vi "nodeInfo.get_OS.vi"(5 "error in (no error)":errorcluster) -> (16 "OS":string, 19 "error out":errorcluster)   [LabVIEW 2014, in "LVNodeInfo.lvlib"]
doc: "Gets the name of the operating system."
uses:
  LVNodeInfo.lvlib
  NodeMon/bin/libNodeInfo.dll
  NodeMon/bin/libNodeInfo.so
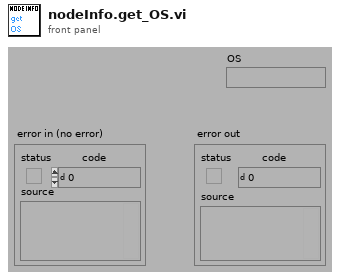
[diagram p1: front panel]
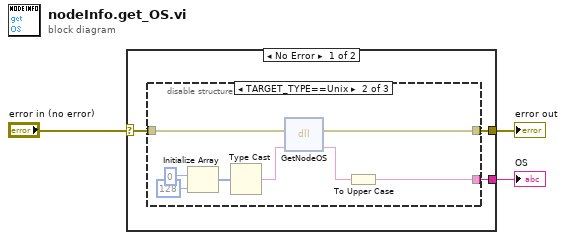
[diagram p0: block diagram]
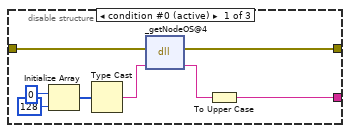
[diagram p2: hidden frame]
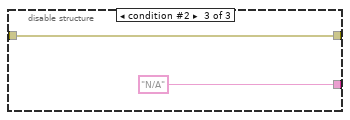
[diagram p3: hidden frame]
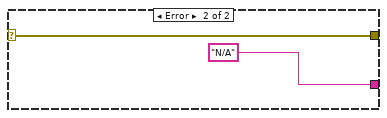
[diagram p4: hidden frame]
diagram:
  n1 = case shown="No Error" "error in (no error)" {
    selector: "error in (no error)" -> [w5 w25]
    tunnel: [w6 "N/A" ("nodeName")] -> w3
    tunnel: [w4 w25] -> w1
    frame No Error {
      n2 = disable-structure "Conditional Disable Structure" shown="TARGET_TYPE==Unix" {
        disable-tunnel: [w9 w17 "N/A"] -> w6
        disable-tunnel: w5 -> [w8 w16 w23]
        disable-tunnel: [w7 w15 w23] -> w4
        frame condition #0 (active) {
          n3 = Initialize Array(i8 0, 128 ("dimension size")) -> (w11:i8[])
          n4 = Type Cast(x=w11) -> (*(type *) &x=w10:string)  [unwired: 1 in]
          n5 = dll-call lib="D:/Git/CS-framework/CSlibraries-extern/DIMLVEvent/NodeMon/bin/libNodeInfo.dll" fn="_getNodeOS@4" label="getNodeOS"(error in=w8, "operatingSystem"=w10) -> (error out=w7:errorcluster, "operatingSystem"=w14:string)  [unwired: 3 in, 1 out]
          n6 = To Upper Case(1:w14) -> (0:w9:string)
        }
        frame condition #1 {
          n7 = Initialize Array(i8 0, 128 ("dimension size")) -> (w19:i8[])
          n8 = Type Cast(x=w19) -> (*(type *) &x=w18:string)  [unwired: 1 in]
          n9 = dll-call lib="D:/Git/CS-framework/CSlibraries-extern/DIMLVEvent/NodeMon/bin/libNodeInfo.so" fn="GetNodeOS"(error in=w16, "operatingSystem"=w18) -> (error out=w15:errorcluster, "operatingSystem"=w22:string)  [unwired: 3 in, 1 out]
          n10 = To Upper Case(1:w22) -> (0:w17:string)
        }
        frame condition #2 {
        }
      }
    }
    frame Error {
    }
  }
  "OS" <- w3
  "error out" <- w1
